vi "Calculate Array Position (SubVI).vi"(6 "Number of Channels":u32, 9 "Elements Remaining":u32, 10 "FIFO Size":u32, 11 "Position":u32) -> (2 "Elements to read":u32, 3 "New Position":u32)   [LabVIEW 2014]
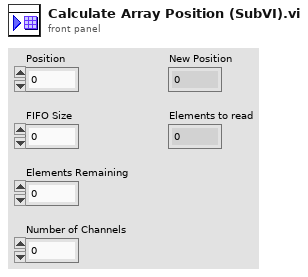
[diagram p1: front panel]
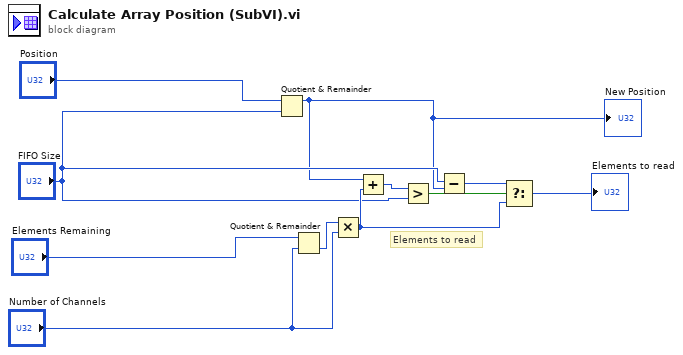
[diagram p0: block diagram]
diagram:
  # "Elements to read"
  n1 = Quotient & Remainder(x="Position", y="FIFO Size") -> (x-y*floor(x/y)=w2:u32)  [unwired: 1 out]
  "New Position" <- w2
  n2 = Quotient & Remainder(x="Elements Remaining", y="Number of Channels") -> (floor(x/y)=w3:u32)  [unwired: 1 out]
  n3 = Multiply(x=w3, y="Number of Channels") -> (x*y=w10:u32)
  n4 = Add(x=w2, y=w10) -> (x+y=w9:u32)
  n5 = Greater?(x=w9, y="FIFO Size") -> (0:w5:bool)
  n6 = Subtract(x="FIFO Size", y=w2) -> (x-y=w7:u32)
  n7 = Select(t=w7, s=w5, f=w10) -> (s? t:f=→"Elements to read":u32)
